vi "Get Current Results.vi"(8 "error in (no error)":errorcluster, 11 "Search in":refnum<class "Search.lvclass">) -> (0 "error out":errorcluster, 2 "Current Results":refnum<class "Search Result.lvclass">[](array[class]), 3 "Search out":refnum<class "Search.lvclass">)   [LabVIEW 2016, in "Better Search.lvlib" / "Search.lvclass"]
uses:
  Search.lvclass
  Search Result/Search Result.lvclass
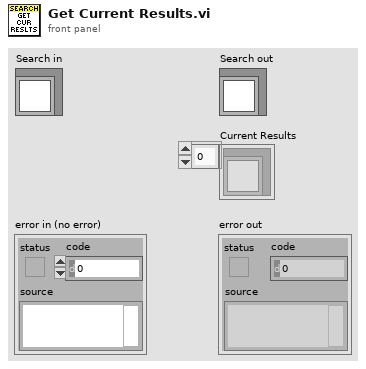
[diagram p1: front panel]
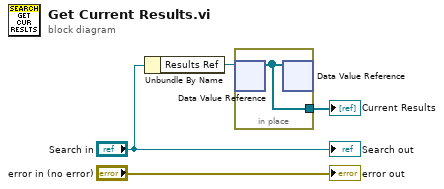
[diagram p0: block diagram]
diagram:
  n1 = Unbundle By Name("Search in") -> ("Results Ref"=w3:refnum<data-value>)
  n2 = in-place {
    in-place-border: [w5] -> w1
    n3 = in-place-dvr #1(w3) -> (w5:refnum<class "Search Result.lvclass">[])  [unwired: 1 out]
    n4 = in-place-dvr #1(w5) -> ()  [unwired: 2 out]
  }
  "Current Results" <- w1
  "error out" <- "error in (no error)"
  "Search out" <- "Search in"
